vi "avoidance test 1.vi"() -> ()   [LabVIEW 2009]
uses:
  object.ctl
  <vilib>/Utility/miscctls.llb/LVPositionTypeDef.ctl
  <vilib>/Utility/miscctls.llb/LVPointTypeDef.ctl
panel:
  in  "Tab":enum32{"draw", "test", "stop"}(tab)
  in  "clear picture":bool
  in  "weight":dbl(slide) min=-10.0 max=10.0 step=0.5 scale=-10.0..10.0
  in  "start point":cluster{"x":i16, "y":i16}
  in  "Speed":sgl(slide) scale=0.0..10.0
  in  "milliseconds to wait":u32(slide) scale=10.0..1000.0
  out "location":cluster{sgl, sgl}
  in  "Array":T1[](array[typedef])
  out "Pic":picture
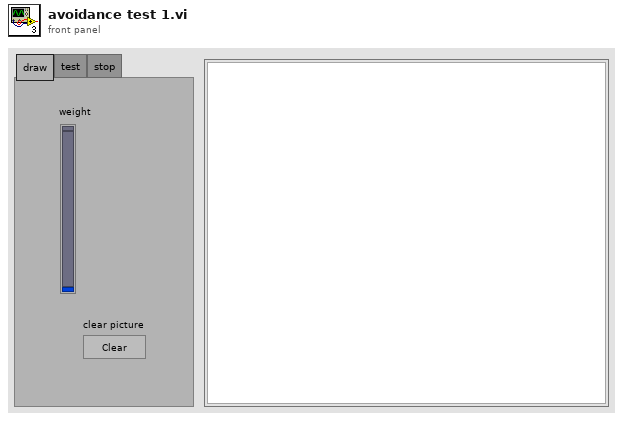
[diagram p1: front panel]
types:
  T1 = typedef "object.ctl" = cluster{"rect":cluster{"left":i16, "top":i16, "right":i16, "bottom":i16}, "weight":sgl}
  T2 = typedef "LVPointTypeDef.ctl" = cluster{"Horizontal":i16, "Vertical":i16}
  T3 = typedef "LVPositionTypeDef.ctl" = cluster{"Left":i32, "Top":i32}
  T4 = cluster{"left":i16, "top":i16, "right":i16, "bottom":i16}
  T5 = typedef "LVPoint32TypeDef.ctl" = cluster{"Horizontal":i32, "Vertical":i32}
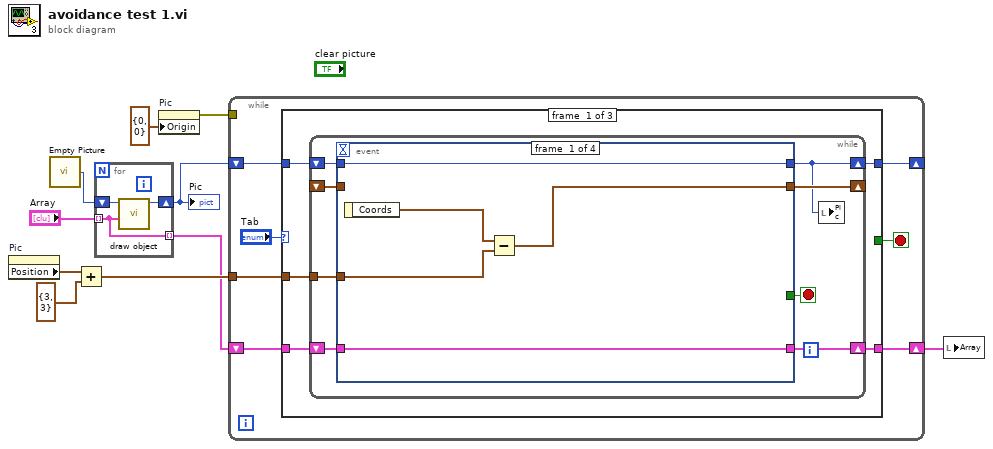
[diagram p0: block diagram]
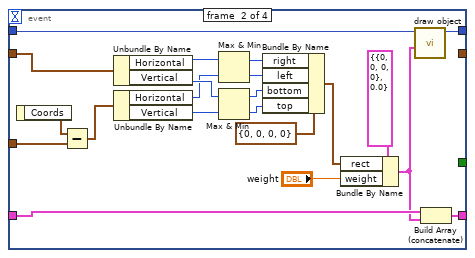
[diagram p2: hidden frame]
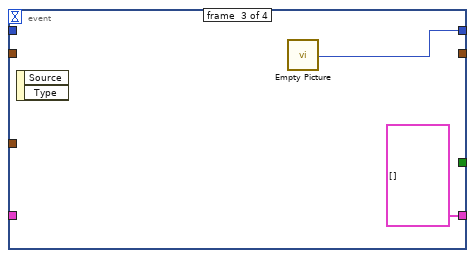
[diagram p3: hidden frame]
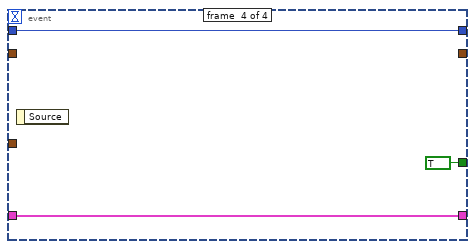
[diagram p4: hidden frame]
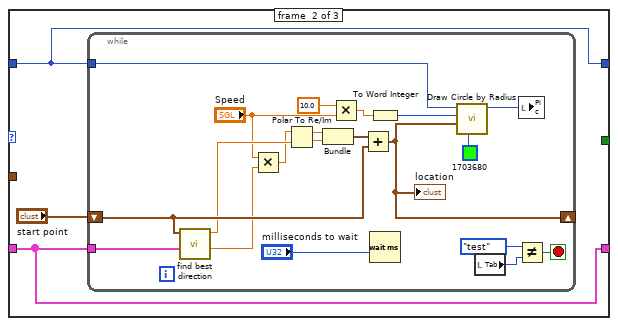
[diagram p5: hidden frame]
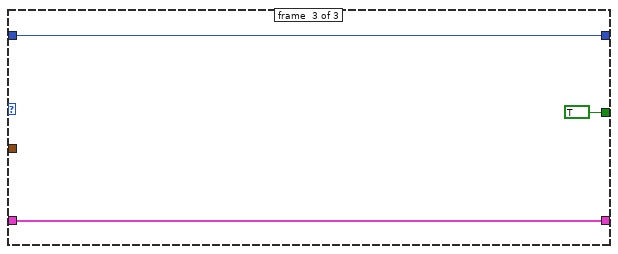
[diagram p6: hidden frame]
diagram:
  n1 = property on="Pic" class="Pict"() -> ("Position"=w10:T3)  [unwired: 2 in, 2 out]
  n2 = call "Empty Picture"() -> ("empty picture"=w2:picture)
  n3 = Add(x=w10, y=T3 {"Left"=3, "Top"=3}) -> (x+y=w7:T3)
  n4 = for {
    tunnel: "Array" -> [w11] mode=indexing
    shift-right: [w13] -> w1
    shift-left: w2 -> [w12]
    tunnel: [w11] -> w3 mode=indexing
    n5 = call "draw object.vi"("Object"=w11, "picture in"=w12) -> ("picture out"=w13:picture)  [unwired: 9 in]
  }
  "Pic" <- w1
  n6 = property on="Pic" class="Pict"("Origin"=T2 {"Horizontal"=0, "Vertical"=0}) -> (error out=w8:errorcluster)  [unwired: 2 in, 1 out]
  n7 = while {
    shift-right: [w20] -> _
    shift-left: w1 -> [w19]
    shift-right: [w16] -> w5
    shift-left: w3 -> [w17]
    tunnel: w8 -> [_]
    tunnel: w7 -> [w14]
    stop <- w15 stop-if-true
    n8 = case shown="\"draw\"" "Tab" {
      tunnel: [w25 w67 w90] -> w20
      tunnel: w19 -> [w24 w67 w90]
      tunnel: w17 -> [w23 w66 w89]
      tunnel: [w22 w66 w89] -> w16
      tunnel: [_ _ TRUE] -> w15
      tunnel: w14 -> [w21 _ _]
      frame #0 {
        n9 = while {
          shift-right: [w33] -> _
          shift-left: _ -> [w32]
          shift-right: [w27] -> w25
          shift-left: w24 -> [w31]
          shift-right: [w28] -> w22
          shift-left: w23 -> [w29]
          tunnel: w21 -> [w26]
          stop <- w30 stop-if-true
          n10 = event shown="[1] \"Pic\": Mouse Up" {
            selector: _ -> [_ _ _ _]
            dyn-events: _ -> [_ _ _ _]
            timeout: _ -> [_ _ _ _]
            tunnel: [w34 _ _ _] -> w33
            tunnel: w32 -> [_ w59 _ _]
            tunnel: [w38 w45 w60 w62] -> w27
            tunnel: w31 -> [w38 w46 _ w62]
            tunnel: [_ _ _ TRUE] -> w30
            tunnel: w29 -> [w37 w49 _ w63]
            tunnel: [w37 w50 T1[] [] w63] -> w28
            tunnel: w26 -> [w35 w42 _ _]
            event #0 {
              n11 = event-data() -> ("Coords"=w36:T5)  [unwired: 1 in]
              n12 = Subtract(x=w36, y=w35) -> (x-y=w34:T5)
            }
            event #1 {
              n13 = event-data() -> ("Coords"=w43:T5)  [unwired: 1 in]
              n14 = Subtract(x=w43, y=w42) -> (x-y=w39:T5)
              n15 = Unbundle By Name(w59) -> ("Horizontal"=w58:i32, "Vertical"=w57:i32)
              n16 = Unbundle By Name(w39) -> ("Horizontal"=w40:i32, "Vertical"=w41:i32)
              n17 = Max & Min(x=w58, y=w40) -> (max(x,y)=w52:i32, min(x,y)=w53:i32)
              n18 = Max & Min(x=w57, y=w41) -> (max(x,y)=w55:i32, min(x,y)=w54:i32)
              n19 = Bundle By Name(cluster=T4 {"left"=0, "top"=0, "right"=0, "bottom"=0} ("rect"), "right"=w52, "left"=w53, "bottom"=w55, "top"=w54) -> (w51:T4)
              n20 = Bundle By Name(cluster=T1 {"rect"={"left"=0, "top"=0, "right"=0, "bottom"=0}, "weight"=0.0} ("Object"), "rect"=w51, "weight"="weight") -> (w44:T1)
              n21 = call "draw object.vi"("Object"=w44, "picture in"=w46) -> ("picture out"=w45:picture)  [unwired: 9 in]
              n22 = Build Array (concatenate)(w49, w44) -> (w50:T1[])
            }
            event #2 {
              n23 = event-data() -> ()  [unwired: 1 in, 2 out]
              n24 = call "Empty Picture"() -> ("empty picture"=w60:picture)
            }
            event #3 {
              n25 = event-data() -> ()  [unwired: 1 in, 1 out]
            }
          }
          n26 = local write "Pic"(w27) -> ()
        }
      }
      frame #1 {
        n27 = while {
          shift-right: [w78] -> _
          shift-left: "start point" -> [w82]
          tunnel: w66 -> [w85]
          tunnel: w67 -> [w76]
          stop <- w74 stop-if-true
          n28 = call "find best direction.vi"("Objects"=w85, "current location"=w82) -> ("magnitude"=w69:sgl, "Direction"=w71:sgl)  [unwired: 8 in]
          n29 = Multiply(x="Speed", y=w69) -> (x*y=w68:sgl)
          n30 = Polar To Re/Im(2:w71, 3:w68) -> (0:w84:sgl, 1:w83:sgl)
          n31 = Bundle(w83, w84) -> (w81:cluster{sgl, sgl})  [unwired: 1 in]
          n32 = Multiply(x=sgl 10.0, y="Speed") -> (x*y=w73:sgl)
          n33 = Add(x=w81, y=w82) -> (x+y=w78:cluster{sgl, sgl})
          "location" <- w78
          n34 = To Word Integer(number=w73) -> (16bit integer=w77:i16)
          n35 = Wait (ms)(milliseconds to wait="milliseconds to wait") -> ()  [unwired: 1 out]
          n36 = call <vilib>:"Draw Circle by Radius.vi"("color(black)"=u32 1703680, "pixel center"=w78, "radius"=w77, "picture"=w76) -> ("new picture"=w75:picture)  [unwired: 7 in]
          n37 = local read "Tab"() -> (w87:enum32{"draw", "test", "stop"})
          n38 = Not Equal?(x=enum32{"draw", "test"}."test", y=w87) -> (x != y?=w74:bool)
          n39 = local write "Pic"(w75) -> ()
        }
      }
      frame #2 {
      }
    }
  }
  n40 = local write "Array"(w5) -> ()
